vi "Text回调.vi"(4 "ValueChange":refnum<user-event>, 5 "事件数据":cluster{"oldValue":string, "newValue":string}, 6 "控件引用":refnum<k24>, 7 "事件通用数据":cluster{"事件源":i32, "事件类型":u32, "时间标识":u32}) -> ()   [LabVIEW 2020]
uses:
  D:/Tyler/Labview/C# Ui/UI/MyTextInput.dll
  UI/MyTextInput.dll
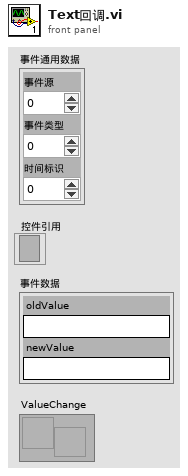
[diagram p1: front panel]
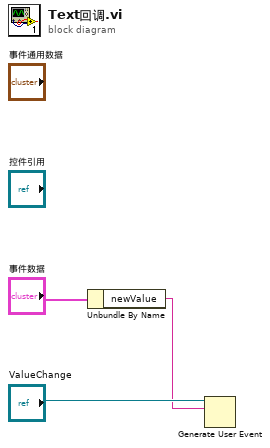
[diagram p0: block diagram]
diagram:
  n1 = Unbundle By Name("事件数据") -> ("newValue"=w1:string)
  n2 = Generate User Event(user event="ValueChange", event data cluster=w1) -> ()  [unwired: 2 in, 2 out]
